vi "StartAcquisitionSD.vi"(2 "error in (no error)":errorcluster) -> (0 "error out":errorcluster, 1 "DLL error code":u32)   [LabVIEW 2015]
doc: "This function starts an acquisition. The status of the acquisition can be monitored via <B>GetStatus</B>.\n\n<B>Error codes:</B>\nDRV_SUCCESS - Acquisition started.\nDRV_NOT_INITIALIZED - System not initialized.\nDRV_ACQUIRING - Acquisition in progress.\nDRV_VXDNOTINSTALLED - VxD not loaded.\nDRV_ERROR_ACK - Unable to communicate with card.\nDRV_INIERROR - Error reading \"DETECTOR.INI\".\nDRV_ACQUISITION_ERRORS - Acquisition settings invalid.\nDRV_ERROR_PAGELOCK - Unable to allocate memory.\nDRV_INVALID_FILTER - Filter not available for current acquisition."
uses:
  DLL/atmcd32d.dll
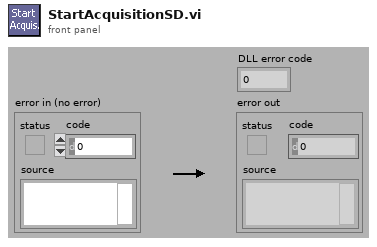
[diagram p1: front panel]
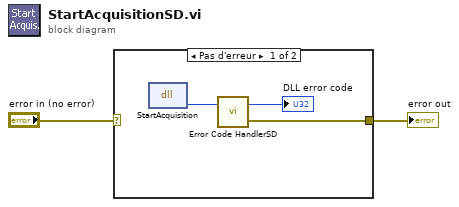
[diagram p0: block diagram]
diagram:
  n1 = case shown="Pas d'erreur" "error in (no error)" {
    selector: "error in (no error)" -> [_ w6]
    tunnel: [w4 w6] -> w1
    frame No Error {
      n2 = dll-call lib="G:/SD/TRANCON/DLL/Atmcd32d.dll" fn="StartAcquisition"() -> (w5:u32)  [unwired: 3 in, 2 out]
      n3 = call "Error Code HandlerSD.vi"("DLL error code"=w5) -> ("error out"=w4:errorcluster, "dup DLL error code"=→"DLL error code":u32)  [unwired: 1 in]
    }
    frame Error {
    }
  }
  "error out" <- w1
